vi "DHE_clear_progress_buf.vi"(0 "fd":i32, 11 "error in (no error)":errorcluster) -> (4 "fd":i32, 8 "return value":i32, 15 "error out":errorcluster)   [LabVIEW 2016]
doc: "This VI closes the I/O interface with the instrument."
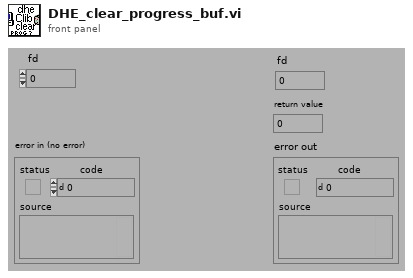
[diagram p1: front panel]
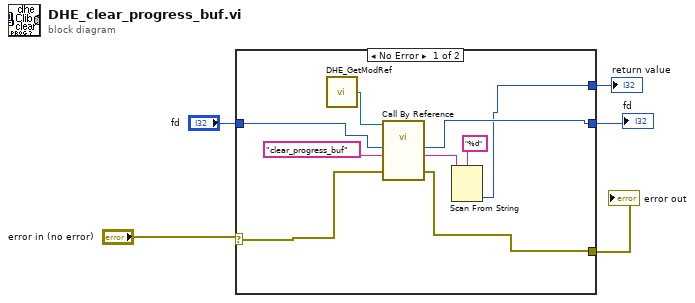
[diagram p0: block diagram]
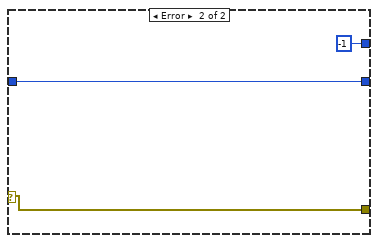
[diagram p2: hidden frame]
diagram:
  n1 = case shown="No Error" "error in (no error)" {
    selector: "error in (no error)" -> [w10 w17]
    tunnel: "fd" -> [w6 w16]
    tunnel: [w9 w17] -> w4
    tunnel: [w8 w16] -> w2
    tunnel: [w7 -1] -> w1
    frame No Error {
      n2 = call "DHE_GetModRef.vi"() -> ("DHE_ModRef"=w14:refnum<vi>)  [unwired: 9 out]
      n3 = call-by-ref "?"(reference=w14, "error in (no error)"=w10, "function"="clear_progress_buf", "fd in"=w6) -> ("error out"=w9:errorcluster, "str result"=w12:string, "fd out"=w8:i32)  [unwired: 6 in, 3 out]
      n4 = Scan From String(format string="%d", input string=w12) -> (output 1=w7:i32)  [unwired: 2 in, 4 out]
    }
    frame Error {
    }
  }
  "error out" <- w4
  "fd" <- w2
  "return value" <- w1
